vi "copy_trading.vi"() -> ()   [LabVIEW 2017]
panel:
  in  "top_trader":bool
  in  "top_profit":bool
  in  "market_based":bool
  in  "Tab Control_main":T1(tab)
  in  "Trading":bool
  in  "Tab Contro_chart":enum32{"chart2"}(tab)
  in  "top_trader1":bool
  in  "top_profit1":bool
  in  "market_based1":bool
  in  "top_trader2":bool
  in  "market_based2":bool
  in  "top_profit2":bool
  in  "mirror1":bool
  in  "top_trader3":bool
  in  "top_profit3":bool
  in  "market_based3":bool
  out "Vertical Fill Slide Indicator":dbl(slide) scale=0.0..100.0
  in  "market_based4":bool
  in  "top_profit4":bool
  in  "top_trader4":bool
  # "-----"
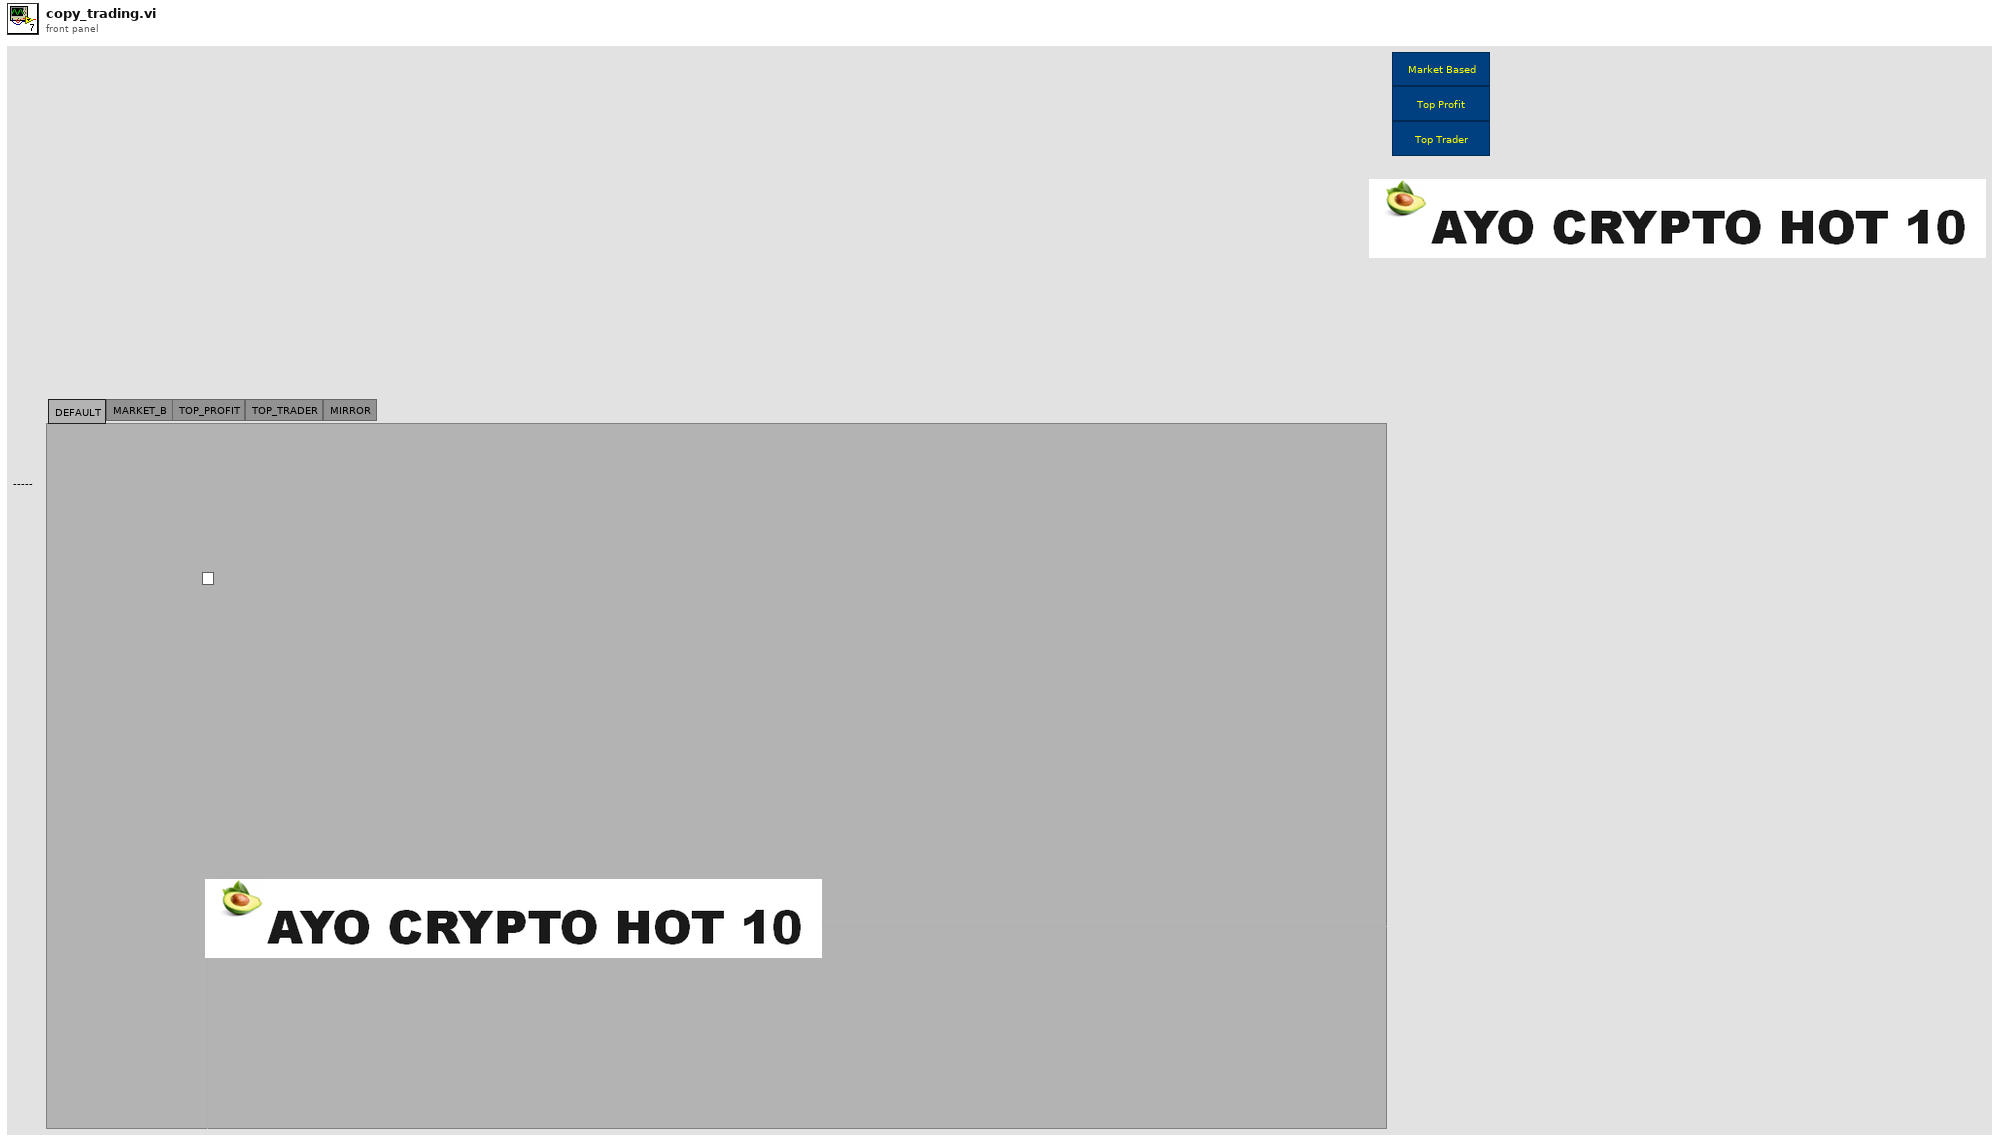
[diagram p1: front panel]
types:
  T1 = enum32{"DEFAULT", "MARKET_B", "TOP_PROFIT", "TOP_TRADER", "MIRROR"}
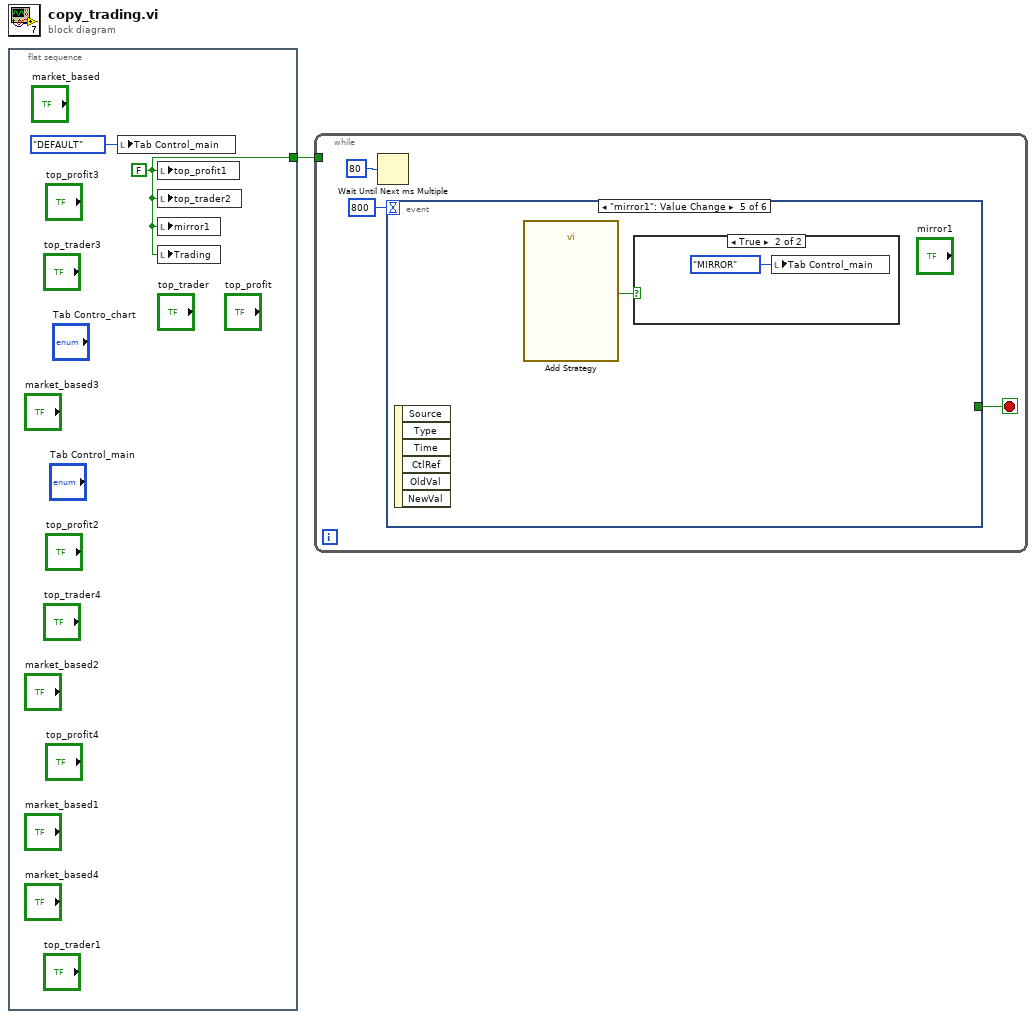
[diagram p0: block diagram]
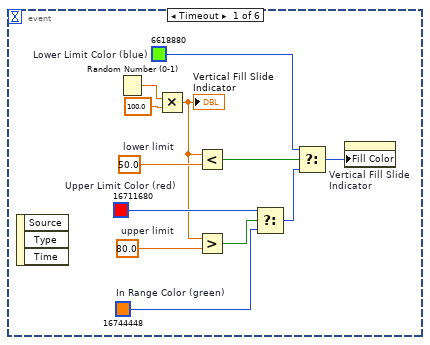
[diagram p2: hidden frame]
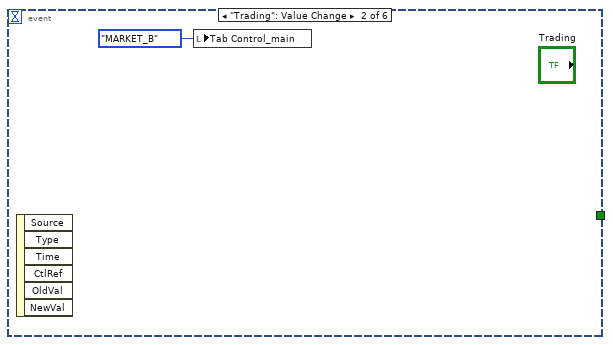
[diagram p3: hidden frame]
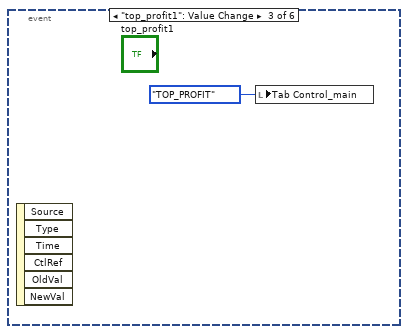
[diagram p4: hidden frame]
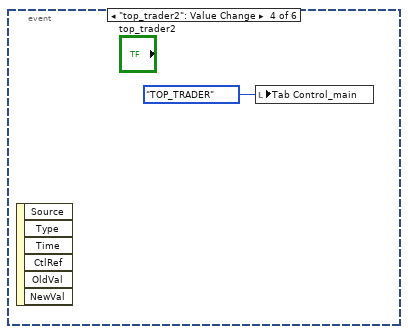
[diagram p5: hidden frame]
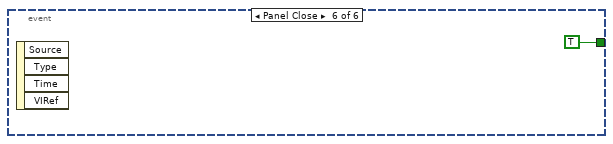
[diagram p7: hidden frame]
diagram:
  n1 = flat-sequence {
    tunnel: [w3] -> w1
    frame #0 {
      w3 = FALSE
      n2 = local write "Tab Control_main"(T1."DEFAULT" ("Tab Control_main")) -> ()
      n3 = local write "top_profit1"(w3) -> ()
      n4 = local write "top_trader2"(w3) -> ()
      n5 = local write "mirror1"(w3) -> ()
      n6 = local write "Trading"(w3) -> ()
    }
  }
  n7 = while {
    tunnel: w1 -> [_]
    stop <- w6 stop-if-true
    n8 = Wait Until Next ms Multiple(millisecond multiple=u32 80) -> ()  [unwired: 1 out]
    n9 = event shown="[4] \"mirror1\": Value Change" {
      selector: _ -> [_ _ _ _ _ _]
      dyn-events: _ -> [_ _ _ _ _ _]
      timeout: 800 -> [_ _ _ _ _ _]
      tunnel: [_ _ _ _ _ TRUE] -> w6
      event Timeout {
        w12 = u32 16744448  # In Range Color (green)
        w9 = u32 6618880  # Lower Limit Color (blue)
        w11 = u32 16711680  # Upper Limit Color (red)
        w10 = 80.0  # upper limit
        w8 = 50.0  # lower limit
        n10 = event-data() -> ()  [unwired: 1 in, 3 out]
        n11 = Random Number (0-1)() -> (number: 0 to 1=w18:dbl)
        n12 = Multiply(x=w18, y=100.0) -> (x*y=w7:dbl)
        "Vertical Fill Slide Indicator" <- w7
        n13 = Less?(x=w7, y=w8) -> (x < y?=w13:bool)
        n14 = Greater?(x=w7, y=w10) -> (0:w14:bool)
        n15 = Select(t=w11, s=w14, f=w12) -> (s? t:f=w15:u32)
        n16 = Select(t=w9, s=w13, f=w15) -> (s? t:f=w16:u32)
        n17 = property on="Vertical Fill Slide Indicator" class="Slide (strict)"("Fill Color"=w16) -> ()  [unwired: 2 in, 2 out]
      }
      event "Trading": Value Change {
        n18 = event-data() -> ()  [unwired: 1 in, 6 out]
        n19 = local write "Tab Control_main"(T1."MARKET_B" ("Tab Control_main")) -> ()
      }
      event "top_profit1": Value Change {
        n20 = event-data() -> ()  [unwired: 1 in, 6 out]
        n21 = local write "Tab Control_main"(T1."TOP_PROFIT" ("Tab Control_main")) -> ()
      }
      event "top_trader2": Value Change {
        n22 = event-data() -> ()  [unwired: 1 in, 6 out]
        n23 = local write "Tab Control_main"(T1."TOP_TRADER" ("Tab Control_main")) -> ()
      }
      event "mirror1": Value Change {
        n24 = event-data() -> ()  [unwired: 1 in, 6 out]
        n25 = call "Add Strategy"() -> ("Add"=w22:bool)  [unwired: 15 in, 4 out]
        n26 = case shown="True" w22 {
          frame False {
          }
          frame True {
            n27 = local write "Tab Control_main"(T1."MIRROR" ("Tab Control_main")) -> ()
          }
        }
      }
      event Panel Close {
        n28 = event-data() -> ()  [unwired: 1 in, 4 out]
      }
    }
  }
